vi "Build Description String.vi"(8 "error in (no error)":errorcluster, 11 "Wait Action in":refnum<class "Wait Action.lvclass">) -> (0 "error out":errorcluster, 2 "Description":string, 3 "Wait Action out":refnum<class "Wait Action.lvclass">)   [LabVIEW 2020, in "MacroAssert.lvlib" / "Wait Action.lvclass"]
doc: "Builds a string to describe what <B>Step</B> does."
uses:
  Wait Action.lvclass
  Action Step/Action Step.lvclass
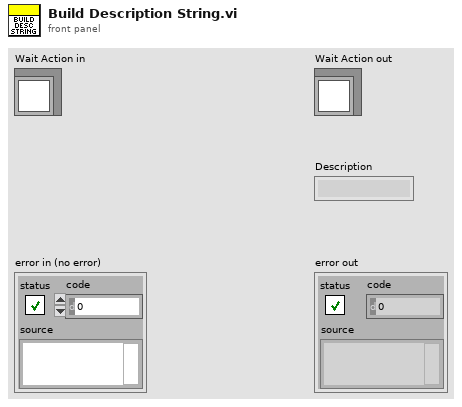
[diagram p1: front panel]
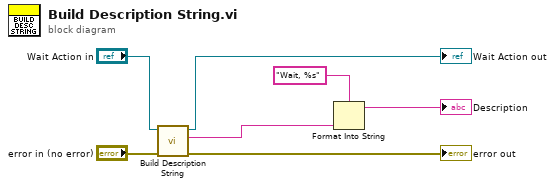
[diagram p0: block diagram]
diagram:
  n1 = call-parent "Build Description String.vi"("error in (no error)"="error in (no error)", "Macro Step in"="Wait Action in") -> ("error out"=→"error out":errorcluster, "Description"=w1:string, "Macro Step out"=→"Wait Action out":refnum<class "Wait Action.lvclass">)  [unwired: 7 in]
  n2 = Format Into String(format string="Wait, %s", w1) -> (resulting string=→"Description":string)  [unwired: 2 in, 1 out]
